vi "Untitled 8 (SubVI).vi"(8 "Reset Integrator":bool, 9 "Temperature (Pure doule precision HW) in":dbl, 10 "Gyroscopic Cluster Values in":cluster{dbl, dbl, dbl}, 11 "Accelorometer Cluster Values in":cluster{i16, i16, i16}) -> (0 "Temperature (Pure doule precision HW) out":dbl, 1 "Linear Acceleration [LSB/sec^2":cluster{i16, i16, i16}, 2 "Angular Displacement (Gyro)":T1, 3 "Angular rate Gyro [LSB/sec]":cluster{dbl, dbl, dbl})   [LabVIEW 2014]
uses:
  <vilib>/ptbypt/NI_PtbyPt.lvlib
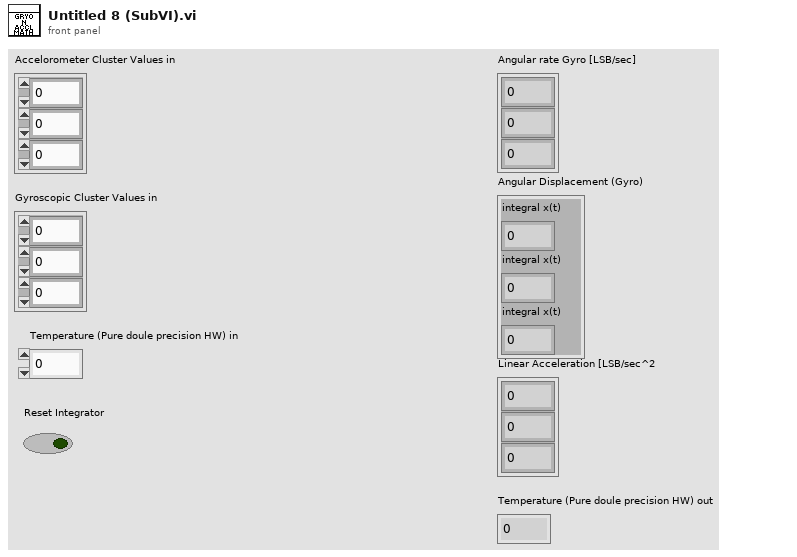
[diagram p1: front panel]
types:
  T1 = cluster{"integral x(t)":dbl, "integral x(t)":dbl, "integral x(t)":dbl}
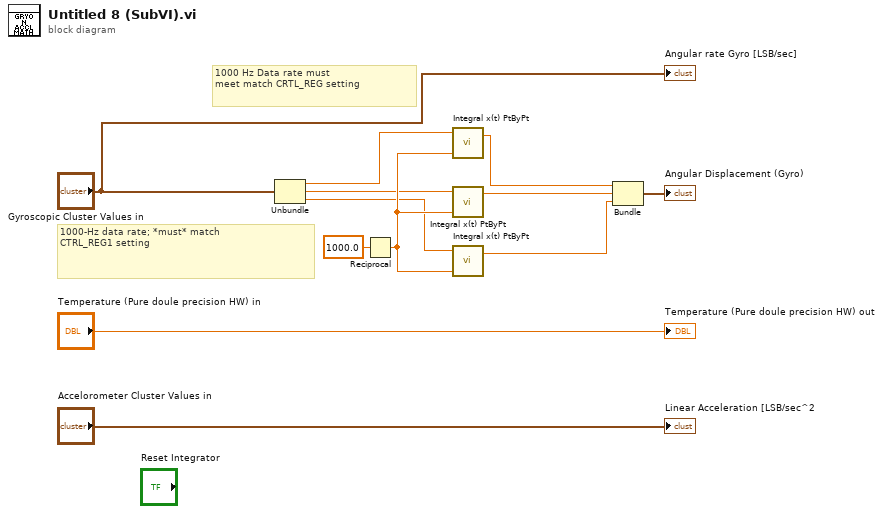
[diagram p0: block diagram]
diagram:
  # "1000 Hz Data rate must\nmeet match CRTL_REG setting"
  # "1000-Hz data rate; *must* match\nCTRL_REG1 setting"
  n1 = Unbundle("Gyroscopic Cluster Values in") -> (w8:dbl, w5:dbl, w4:dbl)
  n2 = Reciprocal(x=1000.0 ("dt")) -> (1/x=w6:dbl)
  n3 = call <vilib>:"Integral x(t) PtByPt.vi"("dt"=w6, "x"=w8) -> ("integral x(t)"=w7:dbl)  [unwired: 2 in, 1 out]
  n4 = call <vilib>:"Integral x(t) PtByPt.vi"("dt"=w6, "x"=w5) -> ("integral x(t)"=w3:dbl)  [unwired: 2 in, 1 out]
  n5 = call <vilib>:"Integral x(t) PtByPt.vi"("dt"=w6, "x"=w4) -> ("integral x(t)"=w2:dbl)  [unwired: 2 in, 1 out]
  n6 = Bundle "Bundle"("integral x(t)"=w7, "integral x(t)"=w3, "integral x(t)"=w2) -> (→"Angular Displacement (Gyro)":T1)  [unwired: 1 in]
  "Linear Acceleration [LSB/sec^2" <- "Accelorometer Cluster Values in"
  "Temperature (Pure doule precision HW) out" <- "Temperature (Pure doule precision HW) in"
  "Angular rate Gyro [LSB/sec]" <- "Gyroscopic Cluster Values in"
